vi "testing_readCoincidence.vi"() -> ()   [LabVIEW 2015, in "Tausand AB1000.lvlib"]
uses:
  <instrlib>/Tausand AB1000/Tausand AB1000.lvlib
  <instrlib>/Tausand AB1000/Public/Controls/deviceTypeRing.ctl
  <instrlib>/Tausand AB1000/Public/Controls/channelRing.ctl
  <vilib>/Analysis/NI_AALBase.lvlib
panel:
  out "num reads":i32
  in  "intervals":i32=20
  out "stddev (s)":dbl format="%0.4f"
  in  "first ch":T1=1 caption="first channel (A=1)" items=["none", "A", "B", "C", "D", "E", "F", "G", "H"]
  in  "second ch":T1=2 caption="second channel (B=2)" items=["none", "A", "B", "C", "D", "E", "F", "G", "H"]
  out "value":u32
  out "label":string
  out "min (s)":dbl format="%0.4f"
  out "max (s)":dbl format="%0.4f"
  out "mean (s)":dbl format="%0.4f"
  out "reading timer histogram":T2(graph)
  in  "stop":bool
  out "last reading timer (s)":dbl format="%0.4f"
  out "error out":errorcluster
  in  "VISA resource name":refnum<visa-resource-name>
  in  "error in (no error)":errorcluster
  out "checksum ok?":bool
  out "read time":timestamp
  in  "read timeout (500 ms)":u32=500
  in  "device type":T3 items=["any"=0, "AB1002"=1002, "AB1004"=1004, "AB1502"=1502, "AB1504"=1504, "AB2002"=2002, "AB2004"=2004, "AB2502"=2502, "AB2504"=2504]
  # "TEST of: 'Read coincidence.vi'"
  # "Reading timer statistics"
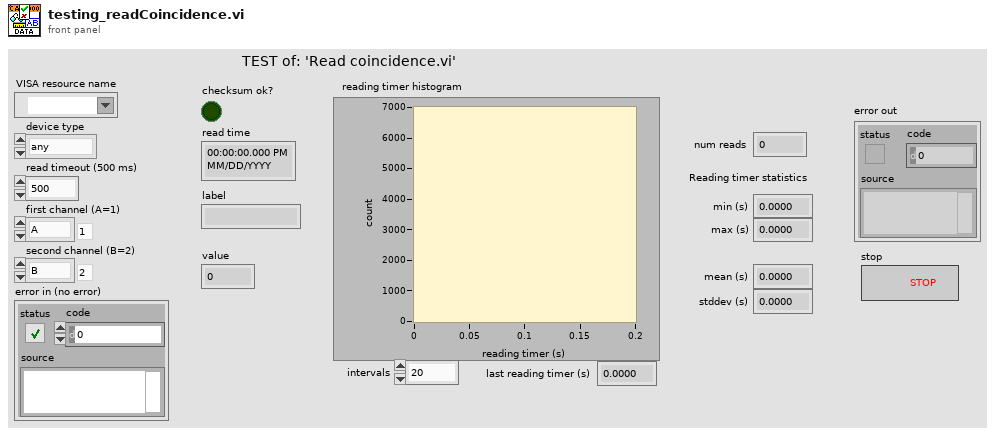
[diagram p1: front panel]
types:
  T1 = typedef "Tausand AB1000.lvlib/channelRing.ctl" = u8
  T2 = cluster{"X Values":dbl[], "Histogram: h(x)":i32[]}
  T3 = typedef "Tausand AB1000.lvlib/deviceTypeRing.ctl" = u16
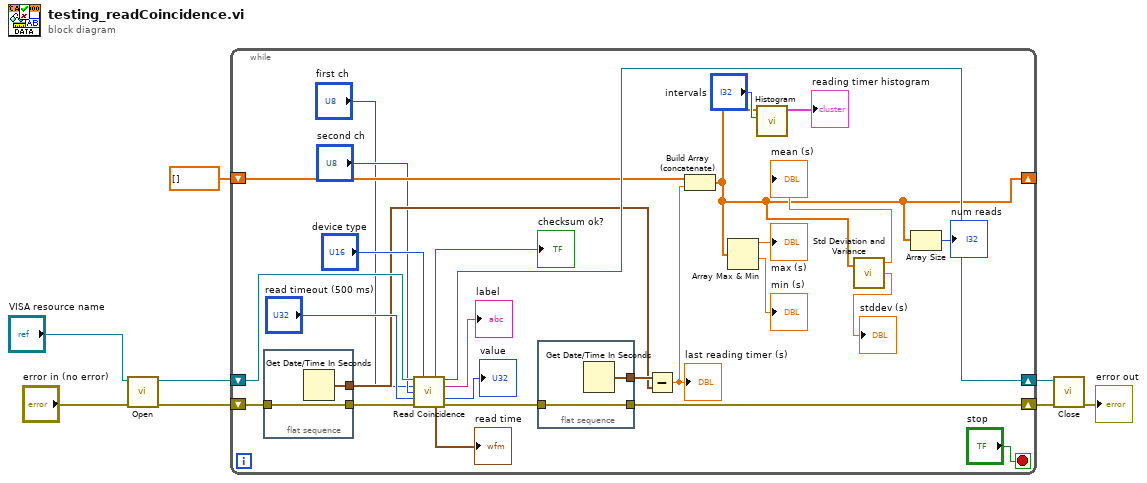
[diagram p0: block diagram]
diagram:
  n1 = call <instrlib>:"Open.vi"("error in (no error)"="error in (no error)", "VISA resource name"="VISA resource name") -> ("error out"=w3:errorcluster, "VISA resource name out"=w8:refnum<visa-resource-name>)  [unwired: 8 in]
  n2 = while {
    shift-right: [w34] -> w7
    shift-left: w8 -> [w35]
    shift-right: [w26] -> w2
    shift-left: w3 -> [w28]
    shift-right: [w10] -> _
    shift-left: dbl[] [] -> [w21]
    stop <- "stop" stop-if-true
    n3 = flat-sequence {
      tunnel: [w39] -> w29
      tunnel: w28 -> [w39]
      tunnel: [w38] -> w24
      frame #0 {
        n4 = Get Date/Time In Seconds() -> (seconds since 1Jan1904=w38:timestamp)
      }
    }
    n5 = call <instrlib>:"Read Coincidence.vi"("VISA Refnum in"=w35, "device type"="device type", "first ch"="first ch", "second ch"="second ch", "read timeout (500 ms)"="read timeout (500 ms)", "error in (no error)"=w29) -> ("checksum ok?"=→"checksum ok?":bool, "VISA Refnum out"=w34:refnum<visa-resource-name>, "label"=→"label":string, "value"=→"value":u32, "read time"=→"read time":timestamp, "error out"=w27:errorcluster)  [unwired: 4 in]
    n6 = flat-sequence {
      tunnel: [w37] -> w26
      tunnel: w27 -> [w37]
      tunnel: [w36] -> w25
      frame #0 {
        n7 = Get Date/Time In Seconds() -> (seconds since 1Jan1904=w36:timestamp)
      }
    }
    n8 = Subtract(x=w25, y=w24) -> (x-y=w22:dbl)
    "last reading timer (s)" <- w22
    n9 = Build Array (concatenate)(w21, w22) -> (w10:dbl[])
    n10 = Array Max & Min(array=w10) -> (max value=→"max (s)":dbl, min value=→"min (s)":dbl)  [unwired: 2 out]
    n11 = call <vilib>:"Histogram.vi"("intervals"="intervals", "X"=w10) -> ("Histogram Graph"=→"reading timer histogram":T2)  [unwired: 6 in, 3 out]
    n12 = call <vilib>:"Std Deviation and Variance.vi"("X"=w10) -> ("mean"=→"mean (s)":dbl, "standard deviation"=→"stddev (s)":dbl)  [unwired: 1 in, 1 out]
    n13 = Array Size(array=w10) -> (size(s)=→"num reads":i32)
  }
  n14 = call <instrlib>:"Close.vi"("error in (no error)"=w2, "VISA resource name"=w7) -> ("error out"=→"error out":errorcluster)  [unwired: 9 in]
